vi "Build Driver Settings Mappings.vi"(8 "error in (no error)":errorcluster, 11 "Driver in":refnum<class "Driver.lvclass">) -> (0 "error out":errorcluster, 2 "Array":T1[](array[typedef]), 3 "Driver out":refnum<class "Driver.lvclass">)   [LabVIEW 2023, in "HAF.lvlib" / "Driver.lvclass"]
uses:
  Driver.lvclass
  Setting Map Structure.ctl
  Driver.lvclass/Driver.ctl
  HAF.lvlib
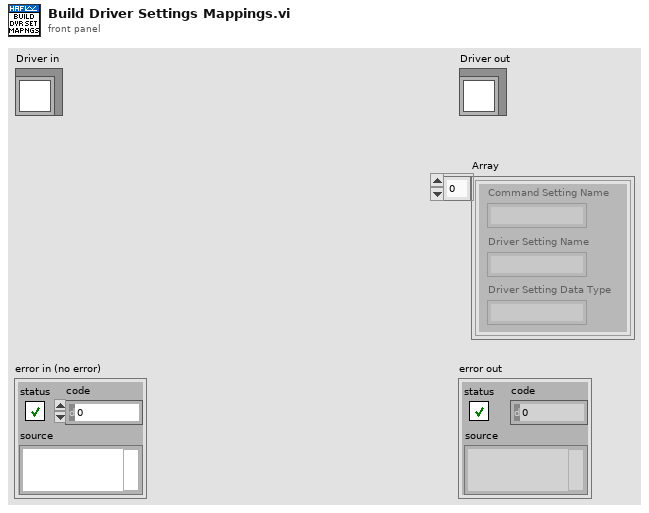
[diagram p1: front panel]
types:
  T1 = typedef "HAF.lvlib/Setting Map Structure.ctl" = cluster{"Command Setting Name":string, "Driver Setting Name":string, "Driver Setting Data Type":string}
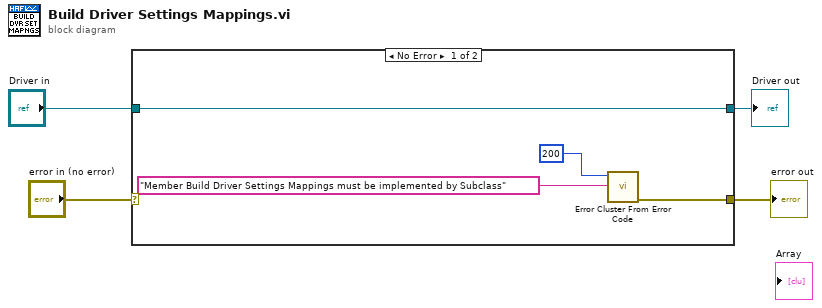
[diagram p0: block diagram]
diagram:
  n1 = case shown="No Error" "error in (no error)" {
    selector: "error in (no error)" -> [_ w10]
    tunnel: [w5 w10] -> w3
    tunnel: [w8 w9] -> w1
    tunnel: "Driver in" -> [w8 w9]
    frame No Error {
      n2 = call <vilib>:"Error Cluster From Error Code.vi"("error message (\"\")"="Member Build Driver Settings Mappings must be implemented by Subclass" ("error message (\"\")"), "error code (0)"=200) -> ("error out"=w5:errorcluster)  [unwired: 7 in]
    }
    frame Error {
    }
  }
  "error out" <- w3
  "Driver out" <- w1
